vi "Make ISD batch file.vi"() -> ()   [LabVIEW 2020]
panel:
  in  "Ports order":i32=1
  in  "ISD":bool
  in  "Open explorer":bool
  out "error out":errorcluster
  out "# of file matches":i32
  out "Filenames":cluster{bool, string}[](array[cluster])
  in  "Test coupon":string="test_coupon"
  out "String":string
  in  "Split 2xThru directly":bool
  in  "Passive":i32=1
  in  "Ports to Skip":i32
  in  "Max Freq (GHz)":dbl=1000.0
  in  "Exit Button":bool
  in  "Save Button":bool
  in  "Test Coupon":T1(ring)=enum."2xThru"
  in  "File name has to include":string
  in  "Test Coupon":path
  in  "Path for snp-files":path
  # "The variable name 2x_thru is\nfollowed by \n1 (default) for “2xThru”, \n2 for “1x Open + 1xShort”, \n3 for “1x Open” or \n4 for “1x Short”."
  # "1 (default) if ports 1 to N are on\nthe left and ports N+1 to 2*N\nare on the right; \n2 if ports 1, 3,5, … are on the left \nand ports 2,4, 6, … are on the right; \n3 if all ports are on the left."
  # "test_coupon\ntest_coupon_open\ntest_coupon_short"
  # "0 (default) for none, \n-1   to skip ports on left\n-2   to skip ports on right\nx    actual indices to skip (such as 1 4 5)"
  # "1 (default) to correct passivity\nand reciprocity for input Touchstone files; \n2 to correct causality; \n3 to correct reciprocity, passivity and causality; \n0 to turn off"
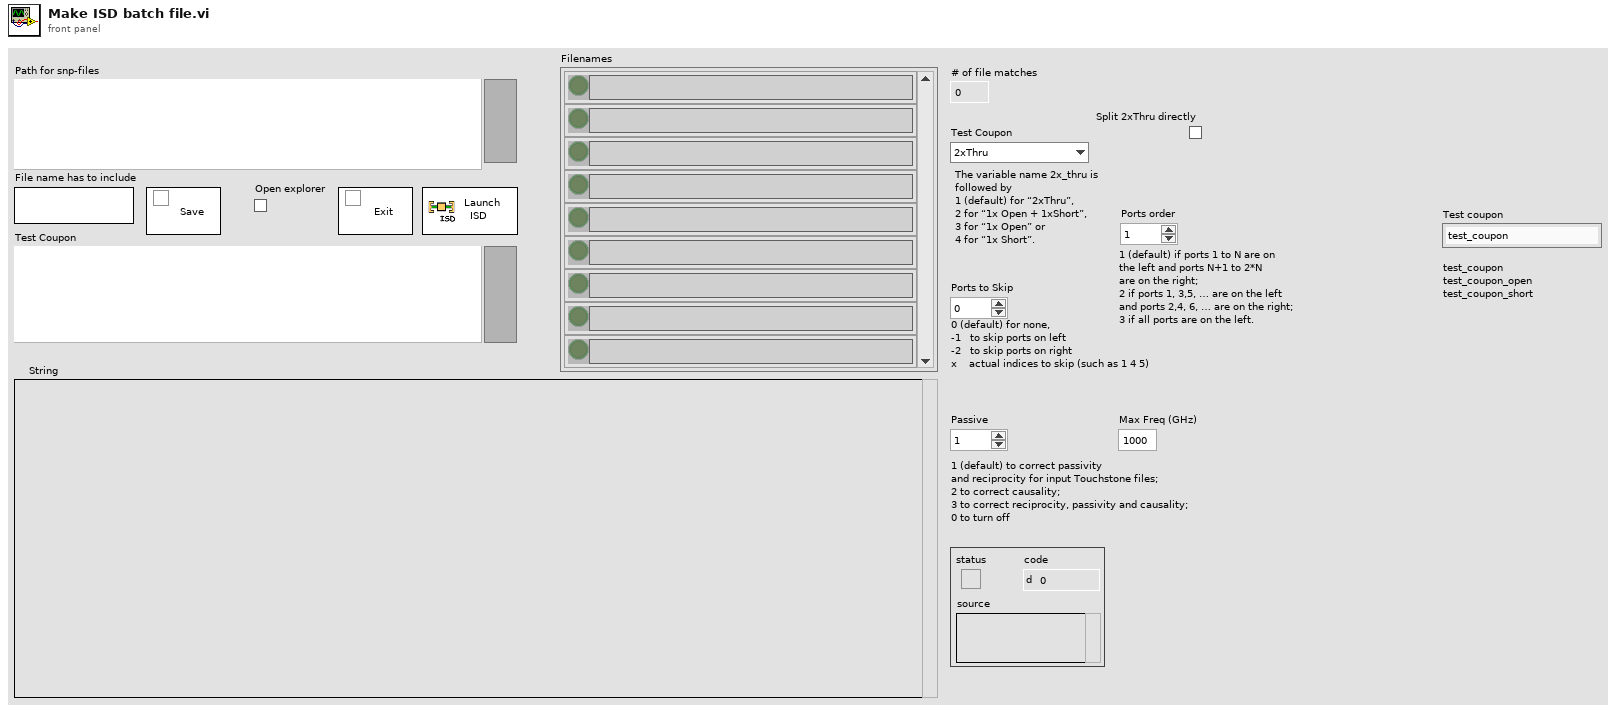
[diagram p1: front panel]
types:
  T1 = enum16{"none", "2xThru", "1xOpen + 1xShort", "1xOpen", "1xshort"}
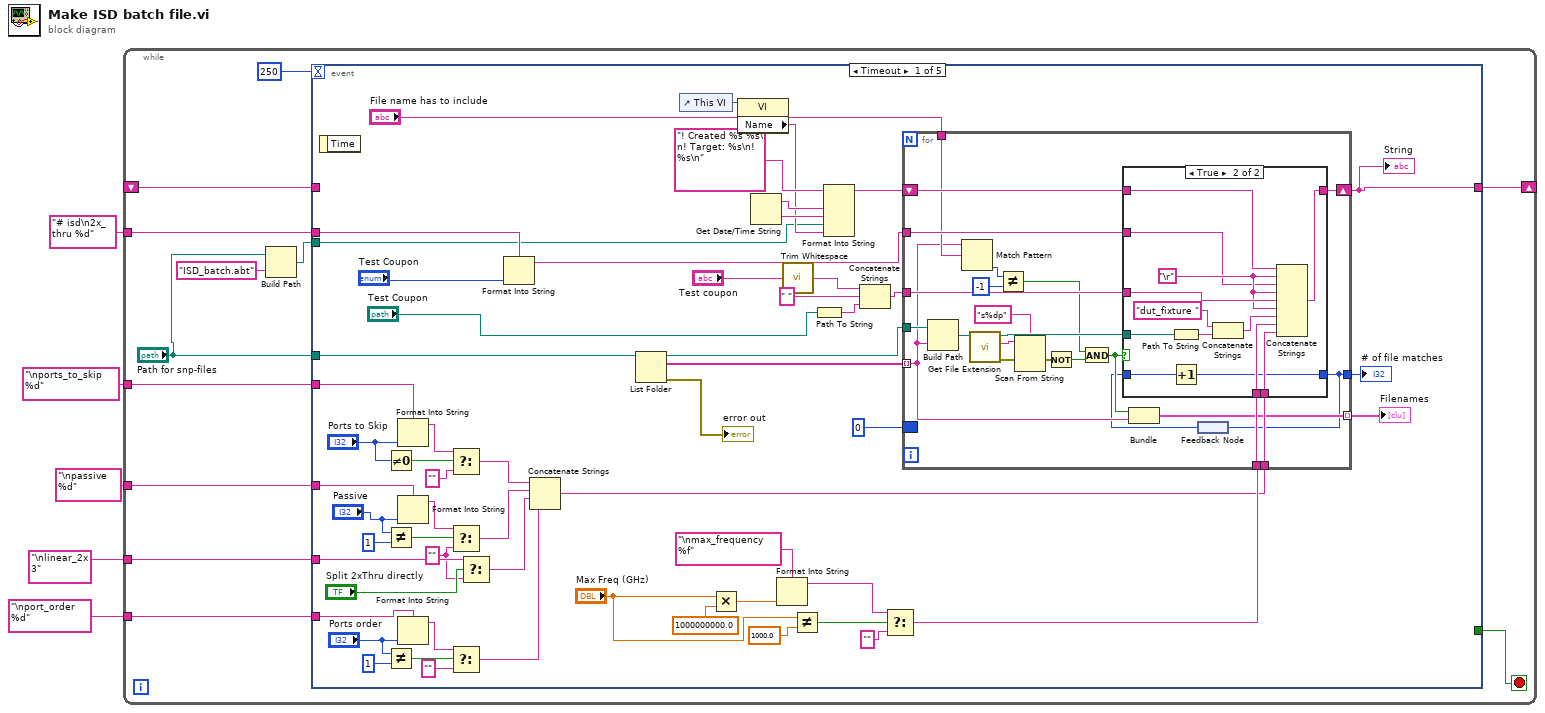
[diagram p0: block diagram]
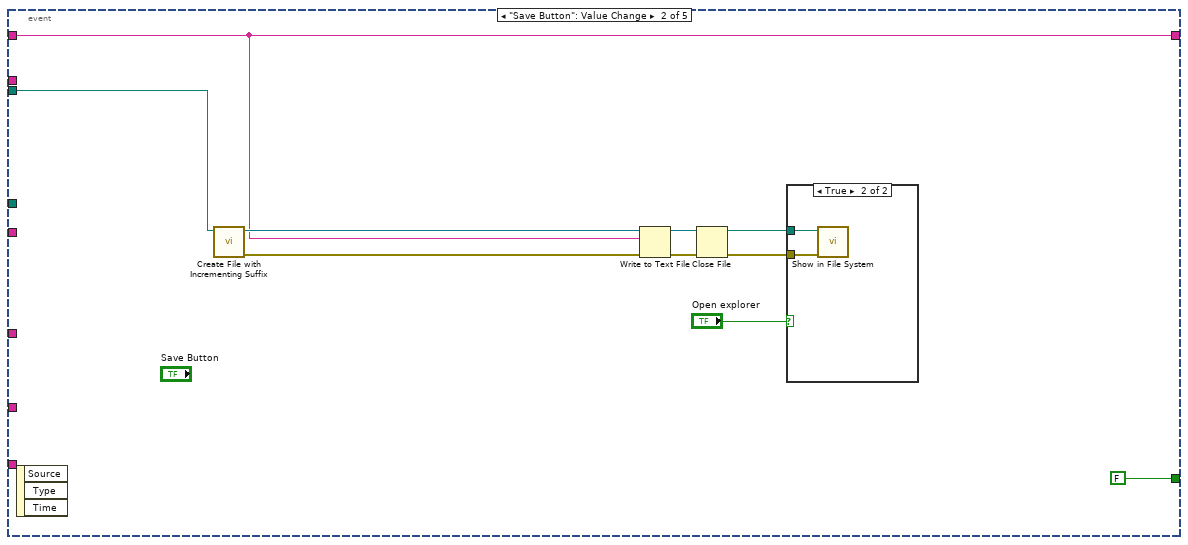
[diagram p3: hidden frame]
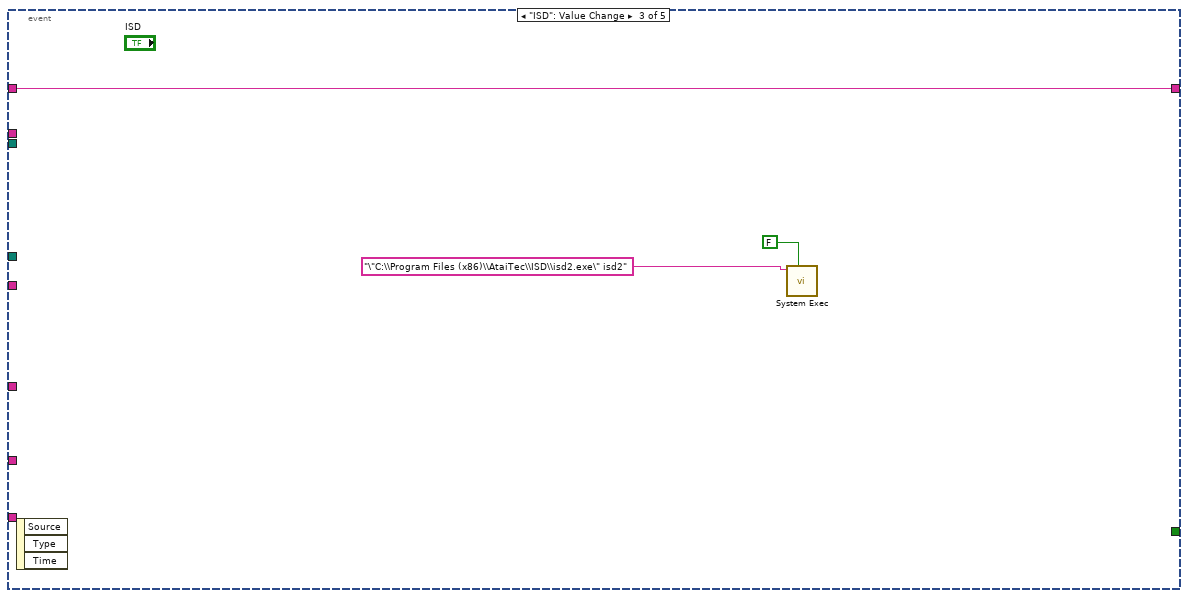
[diagram p5: hidden frame]
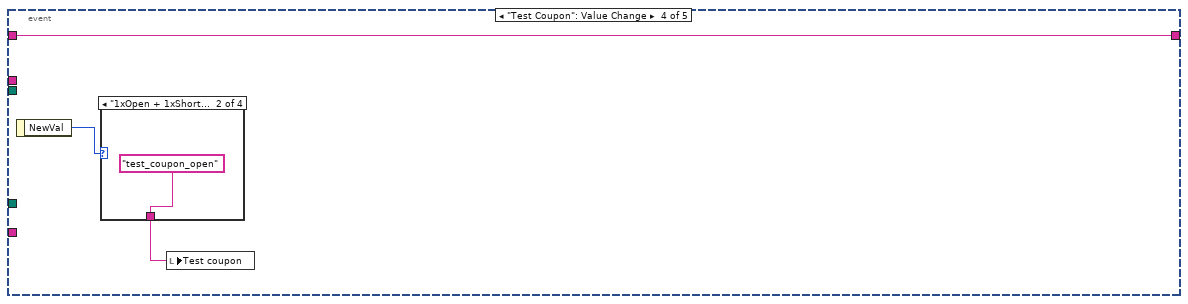
[diagram p6: hidden frame]
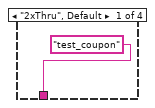
[diagram p7: hidden frame]
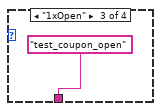
[diagram p8: hidden frame]
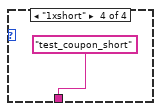
[diagram p9: hidden frame]
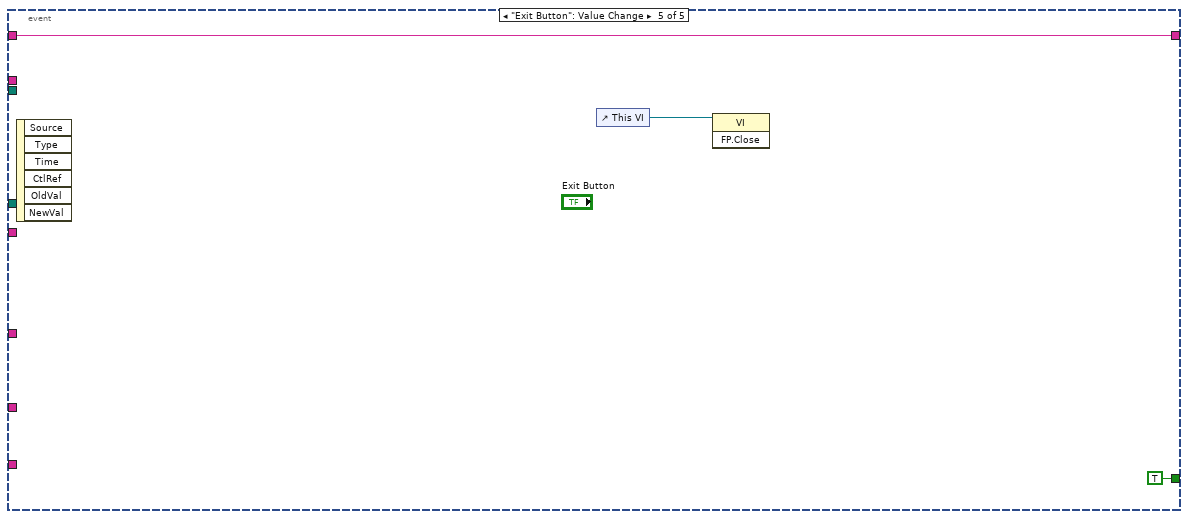
[diagram p10: hidden frame]
diagram:
  n1 = while {
    tunnel: "\npassive %d" ("string") -> [w16]
    tunnel: "\nports_to_skip %d" ("string") -> [w15]
    tunnel: "# isd\n2x_thru %d" ("string") -> [w14]
    tunnel: "\nlinear_2x 3" ("t") -> [w13]
    shift-right: [w8] -> _
    shift-left: _ -> [w7]
    tunnel: "\nport_order %d" ("t") -> [w6]
    stop <- w17 stop-if-true
    n2 = Build Path(base path="Path for snp-files", name or relative path="ISD_batch.abt") -> (appended path=w9:path)
    n3 = event shown="[0] Timeout" {
      selector: _ -> [_ _ _ _ _]
      dyn-events: _ -> [_ _ _ _ _]
      timeout: 250 -> [_ _ _ _ _]
      tunnel: [_ FALSE _ _ TRUE] -> w17
      tunnel: w16 -> [w68 _ _ _ _]
      tunnel: w15 -> [w67 _ _ _ _]
      tunnel: w14 -> [w66 _ _ _ _]
      tunnel: w13 -> [w59 _ _ _ _]
      tunnel: "Path for snp-files" -> [w32 _ _ _ _]
      tunnel: w9 -> [w31 w116 _ _ _]
      tunnel: [w30 w117 w128 w129 w136] -> w8
      tunnel: w7 -> [_ w117 w128 w129 w136]
      tunnel: w6 -> [w21 _ _ _ _]
      event Timeout {
        w58 = "" ("f")
        n4 = event-data() -> ()  [unwired: 1 in, 1 out]
        n5 = Not Equal To 0?(x="Ports to Skip") -> (x != 0?=w73:bool)
        n6 = Not Equal?(x="Passive", y=1 ("x")) -> (x != y?=w69:bool)
        n7 = Not Equal?(x="Ports order", y=1 ("x")) -> (x != y?=w23:bool)
        n8 = Format Into String(format string=w67, "Ports to Skip") -> (resulting string=w71:string)  [unwired: 2 in, 1 out]
        n9 = Format Into String(format string=w68, "Passive") -> (resulting string=w70:string)  [unwired: 2 in, 1 out]
        n10 = Format Into String(format string=w21, "Ports order") -> (resulting string=w22:string)  [unwired: 2 in, 1 out]
        n11 = Select(t=w71, s=w73, f="") -> (s? t:f=w64:string)
        n12 = Select(t=w70, s=w69, f=w58) -> (s? t:f=w65:string)
        n13 = Select(t=w22, s=w23, f="") -> (s? t:f=w19:string)
        n14 = Select(t=w59, s="Split 2xThru directly", f=w58) -> (s? t:f=w61:string)
        n15 = Format Into String(format string=w66, "Test Coupon") -> (resulting string=w36:string)  [unwired: 2 in, 1 out]
        n16 = Concatenate Strings(w64, w65, w61, w19) -> (w33:string)
        n17 = List Folder(path=w32) -> (path out=w57:path, filenames=w28:string[], error out=→"error out":errorcluster)  [unwired: 3 in, 1 out]
        n18 = control-ref of="This VI"() -> (w39:refnum<vi>)
        n19 = Multiply(x="Max Freq (GHz)", y=1000000000.0) -> (x*y=w49:dbl)
        n20 = property class="VI"(reference=w39) -> ("Name"=w38:string)  [unwired: 1 in, 2 out]
        n21 = Get Date/Time String() -> (date string=w40:string, time string=w41:string)  [unwired: 3 in]
        n22 = Format Into String(format string="\nmax_frequency %f" ("string"), w49) -> (resulting string=w46:string)  [unwired: 2 in, 1 out]
        n23 = call <vilib>:"Trim Whitespace.vi"("string"="Test coupon") -> ("trimmed string"=w52:string)  [unwired: 1 in]
        n24 = Not Equal?(x="Max Freq (GHz)", y=1000.0) -> (x != y?=w47:bool)
        n25 = Path To String(path="Test Coupon") -> (string=w56:string)
        n26 = Format Into String(format string="! Created %s %s\n! Target: %s\n! %s\n", w40, w41, w31, w38) -> (resulting string=w42:string)  [unwired: 2 in, 1 out]
        n27 = Concatenate Strings(w52, " " ("string"), w56) -> (w55:string)
        n28 = Select(t=w46, s=w47, f="") -> (s? t:f=w45:string)
        n29 = for {
          tunnel: w28 -> [w84] mode=indexing
          tunnel: w57 -> [w98]
          shift-right: [w96] -> w30
          shift-left: w42 -> [w97]
          tunnel: w55 -> [w95]
          tunnel: w36 -> [w93]
          tunnel: "File name has to include" -> [w92]
          tunnel: w45 -> [w87]
          tunnel: w33 -> [w86]
          tunnel: [w83] -> w29 mode=indexing
          border: 0 -> [_]
          tunnel: [w81] -> w26
          n30 = Build Path(base path=w98, name or relative path=w84) -> (appended path=w88:path)
          n31 = Match Pattern(string=w84, regular expression=w92) -> (offset past match=w91:i32)  [unwired: 1 in, 3 out]
          n32 = call <vilib>:"Get File Extension.vi"("file"=w88) -> ("error out"=w76:errorcluster, "lowercase file extension"=w80:string, "dup file"=w94:path)  [unwired: 6 in, 2 out]
          n33 = Not Equal?(x=w91, y=-1) -> (x != y?=w89:bool)
          n34 = Scan From String(format string="s%dp", input string=w80, error in=w76) -> (error out=w78:errorcluster)  [unwired: 3 in, 2 out]
          n35 = Not(x=w78) -> (.not. x?=w77:bool)
          n36 = And(x=w89, y=w77) -> (x .and. y?=w85:bool)
          n37 = Bundle(w85, w84) -> (w83:cluster{bool, string})  [unwired: 1 in]
          n38 = feedback #1() -> (w82:i32)
          n39 = case shown="True" w85 {
            tunnel: w97 -> [w100 w107]
            tunnel: [w100 w113] -> w96
            tunnel: w95 -> [_ w112]
            tunnel: w94 -> [_ w110]
            tunnel: w93 -> [_ w105]
            tunnel: w87 -> [_ w104]
            tunnel: w86 -> [_ w103]
            tunnel: w82 -> [w99 w101]
            tunnel: [w99 w102] -> w81
            frame False {
            }
            frame True {
              w106 = "\r"
              n40 = Path To String(path=w110) -> (string=w109:string)
              n41 = Increment(x=w101) -> (x+1=w102:i32)
              n42 = Concatenate Strings("dut_fixture " ("string"), w109) -> (w108:string)
              n43 = Concatenate Strings(w107, w106, w105, w106, w112, w106, w108, w104, w103) -> (w113:string)
            }
          }
          n44 = feedback-in #1(w81) -> ()
        }
        "String" <- w30
        "Filenames" <- w29
        "# of file matches" <- w26
      }
      event "Save Button": Value Change {
        n45 = event-data() -> ()  [unwired: 1 in, 3 out]
        n46 = call <vilib>:"Create File with Incrementing Suffix.vi"("file path"=w116) -> ("error out"=w118:errorcluster, "refnum out"=w123:refnum<file>)  [unwired: 8 in, 1 out]
        n47 = Write to Text File(file (use dialog)=w123, text=w117, error in=w118) -> (refnum out=w122:refnum<file>, error out=w119:errorcluster)  [unwired: 1 in, 1 out]
        n48 = Close File(refnum=w122, error in=w119) -> (path=w121:path, error out=w120:errorcluster)
        n49 = case shown="True" "Open explorer" {
          tunnel: w121 -> [_ w125]
          tunnel: w120 -> [_ w124]
          frame False {
          }
          frame True {
            n50 = call <vilib>:"Show in File System.vi"("error in (no error)"=w124, "file or directory path"=w125) -> ()  [unwired: 9 in, 1 out]
          }
        }
      }
      event "ISD": Value Change {
        n51 = event-data() -> ()  [unwired: 1 in, 3 out]
        n52 = call <vilib>:"System Exec.vi"("wait until completion? (T)"=FALSE, "command line"="\"C:\\Program Files (x86)\\AtaiTec\\ISD\\isd2.exe\" isd2") -> ()  [unwired: 6 in, 4 out]
      }
      event "Test Coupon": Value Change {
        n53 = event-data() -> ("NewVal"=w131:T1)  [unwired: 1 in]
        n54 = case shown="\"1xOpen + 1xShort\"" w131 {
          tunnel: ["test_coupon" ("Test coupon") "test_coupon_open" ("Test coupon") "test_coupon_open" ("Test coupon") "test_coupon_short" ("Test coupon")] -> w130
          frame "2xThru", Default {
          }
          frame "1xOpen + 1xShort" {
          }
          frame "1xOpen" {
          }
          frame "1xshort" {
          }
        }
        n55 = local write "Test coupon"(w130) -> ()
      }
      event "Exit Button": Value Change {
        n56 = event-data() -> ()  [unwired: 1 in, 6 out]
        n57 = control-ref of="This VI"() -> (w137:refnum<vi>)
        n58 = invoke class="VI" method="FP.Close"(reference=w137) -> ()  [unwired: 2 in, 3 out]
      }
    }
  }
